vi "Inspect BBM Pad Groups.vi"(7 "Console Log in":refnum<class "Console Log.lvclass">, 8 "error in":errorcluster, 10 "Module Data In":T1={"TBM-TBM"={"Fiducial Image"={"Image Position"=refnum, "Image Reference"=refnum, "Field of View"={"x(mm)"=0.0, "y(mm)"=0.0}}, "Fiducials"=[]}, "TBM-HDI"={"Fiducial Image"={"Image Position"=refnum, "Image Reference"=refnum, "Field of View"={"x(mm)"=0.0, "y(mm)"=0.0}}, "Fiducials"=[]}, "Address Pads"={"Fiducial Image"={"Image Position"=refnum, "Image Reference"=refnum, "Field of View"={"x(mm)"=0.0, "y(mm)"=0.0}}, "Fiducials"=[]}, "HDI Bond Pad References"=[], "BBM Bond Pad References"=[], "HV-HDI"={"Fiducial Image"={"Image Position"=refnum, "Image Reference"=refnum, "Field of View"={"x(mm)"=0.0, "y(mm)"=0.0}}, "Selected Fiducial"={"Fiducial Image Coordinate"=refnum, "Fiducial Source"=enum."Pattern Recognition"}, "fiducial name"=""}, "HV-BBM"={"Fiducial Image"={"Image Position"=refnum, "Image Reference"=refnum, "Field of View"={"x(mm)"=0.0, "y(mm)"=0.0}}, "Selected Fiducial"={"Fiducial Image Coordinate"=refnum, "Fiducial Source"=enum."Pattern Recognition"}, "fiducial name"=""}, "Chuck"=0, "Slot"=0, "Potting Selection"={"HDI Bond Pads"=[TRUE, TRUE, TRUE, TRUE, TRUE, TRUE, TRUE, TRUE, TRUE, TRUE, TRUE, TRUE, TRUE, TRUE, TRUE, TRUE], "BBM Bond Pads"=[TRUE, TRUE, TRUE, TRUE, TRUE, TRUE, TRUE, TRUE, TRUE, TRUE, TRUE, TRUE, TRUE, TRUE, TRUE, TRUE], "TBM Inner"={"Top"=TRUE, "Left"=TRUE, "Bottom"=TRUE, "Right"=TRUE}, "TBM Outer"={"Top"=TRUE, "Left"=TRUE, "Bottom"=TRUE, "Right"=TRUE}, "Address Pads"={"Top"=TRUE, "Bottom"=TRUE}, "High Voltage"={"HDI"=TRUE, "Sensor"=TRUE}}}, 11 "Potting Procedure in":refnum<class "Potting Procedure.lvclass">) -> (0 "error out":errorcluster, 2 "Module Data Out":T1={"TBM-TBM"={"Fiducial Image"={"Image Position"=refnum, "Image Reference"=refnum, "Field of View"={"x(mm)"=0.0, "y(mm)"=0.0}}, "Fiducials"=[]}, "TBM-HDI"={"Fiducial Image"={"Image Position"=refnum, "Image Reference"=refnum, "Field of View"={"x(mm)"=0.0, "y(mm)"=0.0}}, "Fiducials"=[]}, "Address Pads"={"Fiducial Image"={"Image Position"=refnum, "Image Reference"=refnum, "Field of View"={"x(mm)"=0.0, "y(mm)"=0.0}}, "Fiducials"=[]}, "HDI Bond Pad References"=[], "BBM Bond Pad References"=[], "HV-HDI"={"Fiducial Image"={"Image Position"=refnum, "Image Reference"=refnum, "Field of View"={"x(mm)"=0.0, "y(mm)"=0.0}}, "Selected Fiducial"={"Fiducial Image Coordinate"=refnum, "Fiducial Source"=enum."Pattern Recognition"}, "fiducial name"=""}, "HV-BBM"={"Fiducial Image"={"Image Position"=refnum, "Image Reference"=refnum, "Field of View"={"x(mm)"=0.0, "y(mm)"=0.0}}, "Selected Fiducial"={"Fiducial Image Coordinate"=refnum, "Fiducial Source"=enum."Pattern Recognition"}, "fiducial name"=""}, "Chuck"=0, "Slot"=0, "Potting Selection"={"HDI Bond Pads"=[TRUE, TRUE, TRUE, TRUE, TRUE, TRUE, TRUE, TRUE, TRUE, TRUE, TRUE, TRUE, TRUE, TRUE, TRUE, TRUE], "BBM Bond Pads"=[TRUE, TRUE, TRUE, TRUE, TRUE, TRUE, TRUE, TRUE, TRUE, TRUE, TRUE, TRUE, TRUE, TRUE, TRUE, TRUE], "TBM Inner"={"Top"=TRUE, "Left"=TRUE, "Bottom"=TRUE, "Right"=TRUE}, "TBM Outer"={"Top"=TRUE, "Left"=TRUE, "Bottom"=TRUE, "Right"=TRUE}, "Address Pads"={"Top"=TRUE, "Bottom"=TRUE}, "High Voltage"={"HDI"=TRUE, "Sensor"=TRUE}}}, 3 "Potting Procedure out":refnum<class "Potting Procedure.lvclass">, 5 "Console Log out":refnum<class "Console Log.lvclass">)   [LabVIEW 2011, in "Potting Procedure.lvclass"]
uses:
  Potting Procedure.lvclass
  UI Classes/Console Log/Console Log.lvclass
  Type Definitions/Inspect Modules - Module.ctl
  Shared Components/Vec3d Class/Vec3d Class.lvclass
  Shared Components/Utils/Type Definitions/Multi-Fiducial Image.ctl
  Shared Components/Utils/Type Definitions/Physical Image.ctl
  <vilib>/vision/Image Controls.llb/IMAQ Image.ctl
  Shared Components/Utils/Type Definitions/Fiducial with Source.ctl
  Shared Components/Utils/Type Definitions/Fiducial Image.ctl
  Shared Components/WorkTable Class/WorkTable Class.lvclass
  Shared Components/Gantry Class/Gantry Class.lvclass
  Shared Components/Config Manager Class/Type Definitions/Part Type.ctl
  Shared Components/Config Manager Class/Read Geometry Definition 3D.vi
  Shared Components/Config Manager Class/Config Manager Class.lvclass
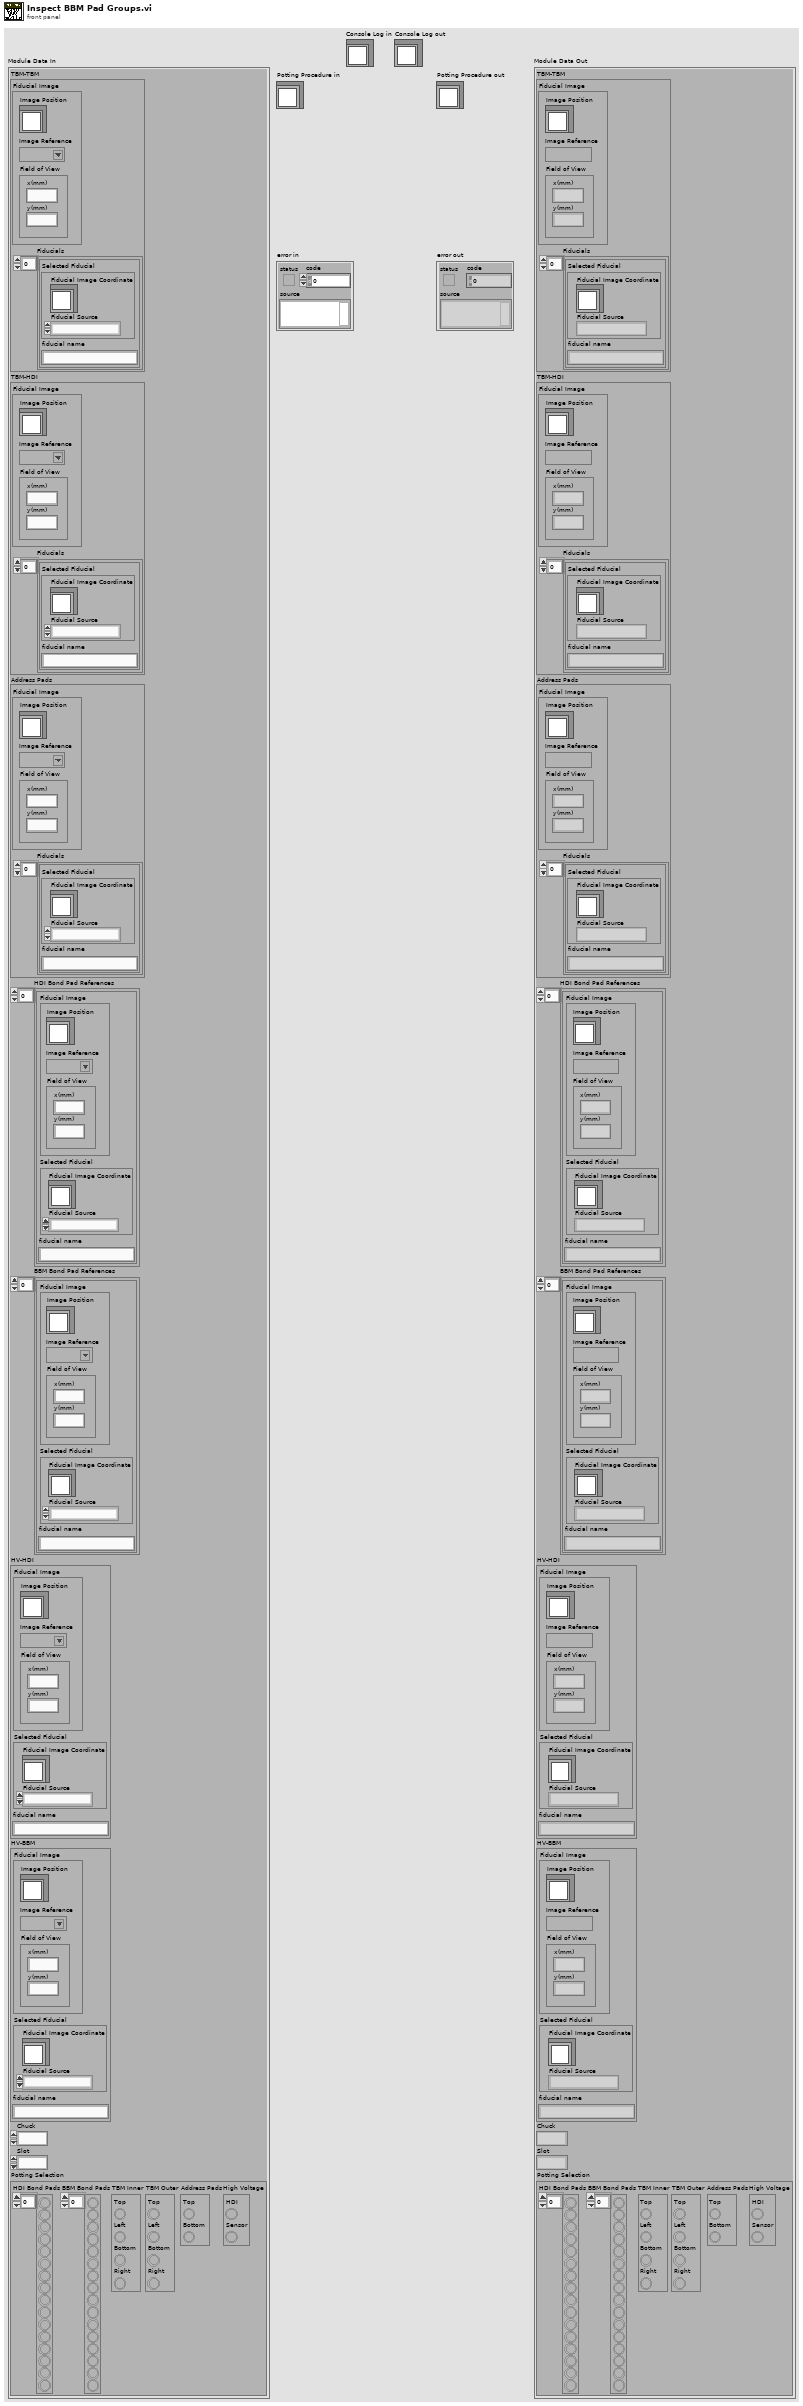
[diagram p1: front panel]
types:
  T1 = typedef "Inspect Modules - Module.ctl" = cluster{"TBM-TBM":T2, "TBM-HDI":T2, "Address Pads":T2, "HDI Bond Pad References":T6[], "BBM Bond Pad References":T6[], "HV-HDI":T6, "HV-BBM":T6, "Chuck":i32, "Slot":i32, "Potting Selection":cluster{"HDI Bond Pads":bool[], "BBM Bond Pads":bool[], "TBM Inner":cluster{"Top":bool, "Left":bool, "Bottom":bool, "Right":bool}, "TBM Outer":cluster{"Top":bool, "Left":bool, "Bottom":bool, "Right":bool}, "Address Pads":cluster{"Top":bool, "Bottom":bool}, "High Voltage":cluster{"HDI":bool, "Sensor":bool}}}
  T2 = typedef "Multi-Fiducial Image.ctl" = cluster{"Fiducial Image":T3, "Fiducials":cluster{"Selected Fiducial":T5, "fiducial name":string}[]}
  T3 = typedef "Physical Image.ctl" = cluster{"Image Position":refnum<class "Vec3d Class.lvclass">, "Image Reference":T4, "Field of View":cluster{"x(mm)":dbl, "y(mm)":dbl}}
  T4 = typedef "IMAQ Image.ctl" = refnum<image>
  T5 = typedef "Fiducial with Source.ctl" = cluster{"Fiducial Image Coordinate":refnum<class "Vec3d Class.lvclass">, "Fiducial Source":enum16{"Pattern Recognition", "User", "Error", "Default"}}
  T6 = typedef "Fiducial Image.ctl" = cluster{"Fiducial Image":T3, "Selected Fiducial":T5, "fiducial name":string}
  T7 = typedef "Part Type.ctl" = enum16{"BBM", "HDI", "GLUERESERVOIR", "STAMP", "WEIGHT"}
  T8 = enum16{"Pattern Recognition", "User", "Error", "Default"}
  T9 = typedef "Worktable_Module Slot.ctl" = cluster{"Slot State":enum16{"Empty", "Unglued", "Stamped", "PartOnTop", "Weighted", "Unpotted", "Potted"}, "BBM Type":enum16{"None", "BBM", "GlassSlide"}, "HDI Type":enum16{"None", "HDI", "Polyimide"}, "Vacuum Channel":u8, "Location/Orientation BBM":T10, "Location/Orientation HDI":T10, "S/N":string}
  T10 = typedef "Position_Orientation.ctl" = cluster{"Center":refnum<class "Vec3d Class.lvclass">, "Orientation":refnum<class "Orient3d Class.lvclass">}
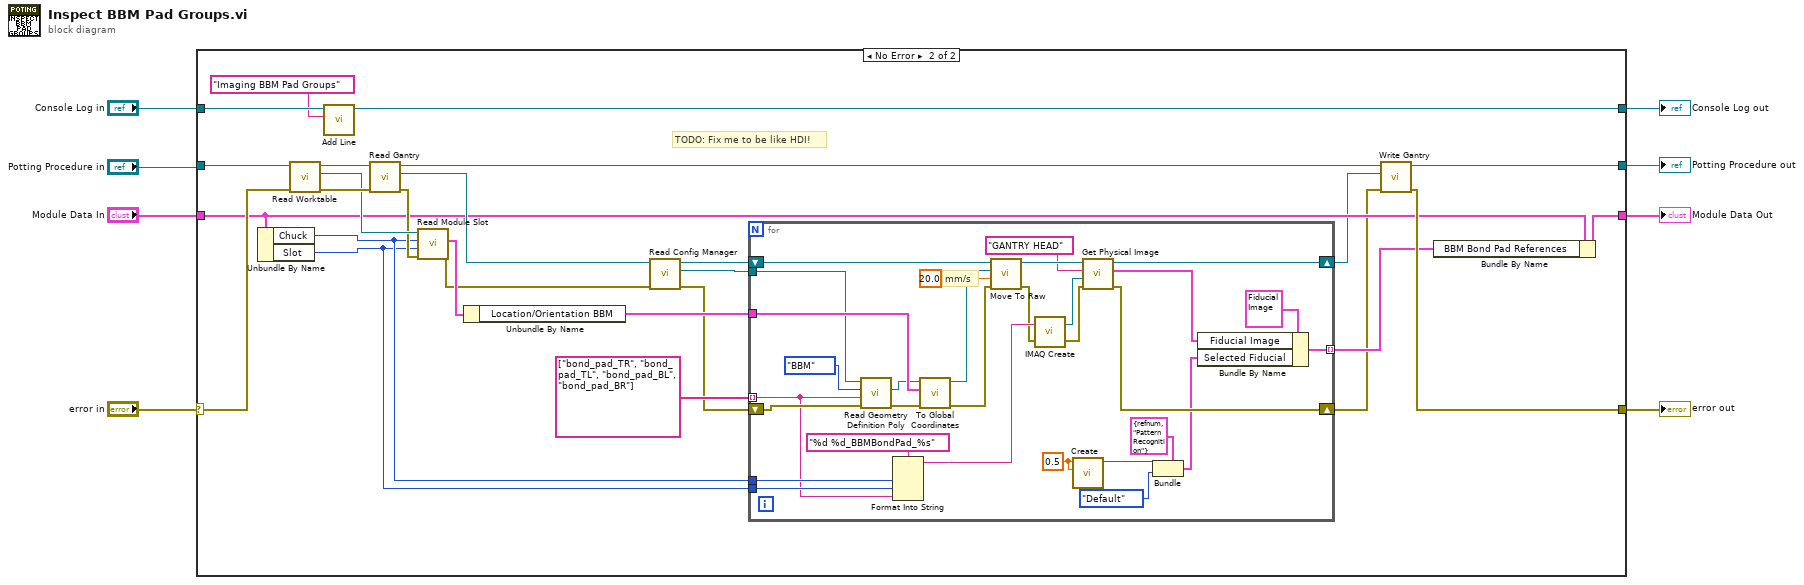
[diagram p0: block diagram]
diagram:
  n1 = case shown="No Error" "error in" {
    selector: "error in" -> [w11 w37]
    tunnel: [w11 w27] -> w6
    tunnel: [w12 w28] -> w5
    tunnel: "Potting Procedure in" -> [w12 w39]
    tunnel: "Module Data In" -> [w10 w26]
    tunnel: [w10 w30] -> w1
    tunnel: "Console Log in" -> [w9 w25]
    tunnel: [w9 w23] -> w3
    frame Error {
    }
    frame No Error {
      # "TODO: Fix me to be like HDI!"
      n2 = Unbundle By Name(w26) -> ("Chuck"=w18:i32, "Slot"=w17:i32)
      n3 = call-dynamic "Read Worktable.vi"("error in"=w37, "Potting Procedure in"=w39) -> ("error out"=w36:errorcluster, "WorkTable out"=w35:refnum<class "WorkTable Class.lvclass">, "Potting Procedure out"=w38:refnum<class "Potting Procedure.lvclass">)  [unwired: 7 in]
      n4 = call "Add Line.vi"("String"="Imaging BBM Pad Groups", "Console Log in"=w25) -> ("Console Log out"=w23:refnum<class "Console Log.lvclass">)  [unwired: 8 in, 1 out]
      n5 = call-dynamic "Read Gantry.vi"("error in (no error)"=w36, "Potting Procedure in"=w38) -> ("error out"=w34:errorcluster, "Gantry"=w32:refnum<class "Gantry Class.lvclass">, "Potting Procedure out"=w29:refnum<class "Potting Procedure.lvclass">)  [unwired: 7 in]
      n6 = call-dynamic "Read Module Slot.vi"("error in"=w34, "slot"=w17, "chuck"=w18, "WorkTable in"=w35) -> ("error out"=w31:errorcluster, "Module Slot"=w33:T9)  [unwired: 5 in, 1 out]
      n7 = Unbundle By Name(w33) -> ("Location/Orientation BBM"=w20:T10)
      n8 = call-dynamic "Read Config Manager.vi"("error in"=w31, "Gantry in"=w32) -> ("error out"=w13:errorcluster, "Config Manager"=w21:refnum<class "Config Manager Class.lvclass">, "Gantry out"=w22:refnum<class "Gantry Class.lvclass">)  [unwired: 7 in]
      n9 = for {
        tunnel: string[] ["bond_pad_TR", "bond_pad_TL", "bond_pad_BL", "bond_pad_BR"] -> [w42] mode=indexing
        tunnel: w20 -> [w69]
        shift-right: [w54] -> w15
        shift-left: w13 -> [w43]
        tunnel: w18 -> [w62]
        tunnel: w17 -> [w61]
        shift-right: [w55] -> w14
        shift-left: w22 -> [w68]
        tunnel: [w46] -> w16 mode=indexing
        tunnel: w21 -> [w45]
        w48 = 0.5 ("X")
        # "mm/s"
        n10 = call-poly "Read Geometry Definition Poly.vi"("error in"=w43, "Feature"=w42, "Part Type"=Part_Type."BBM", "Config Manager in"=w45) -> ("error out"=w40:errorcluster, "Feature Coordinates"=w41:refnum<class "Vec3d Class.lvclass">)  [unwired: 5 in, 1 out]
        n11 = Format Into String(format string="%d %d_BBMBondPad_%s", w62, w61, w42) -> (resulting string=w60:string)  [unwired: 2 in, 1 out]
        n12 = call "To Global Coordinates.vi"("error in"=w40, "Center/Orientation"=w69, "Local Coordinates"=w41) -> ("error out"=w65:errorcluster, "Global Coordinates"=w67:refnum<class "Vec3d Class.lvclass">)  [unwired: 7 in]
        n13 = call-dynamic "Move To Raw.vi"("error in"=w65, "Speed"=20.0, "Destination"=w67, "Gantry in"=w68) -> ("error out"=w59:errorcluster, "Gantry out"=w64:refnum<class "Gantry Class.lvclass">)  [unwired: 6 in]
        n14 = call "IMAQ Create"("Image Name"=w60, "error in (no error)"=w59) -> ("New Image"=w57:T4, "error out"=w58:errorcluster)  [unwired: 3 in]
        n15 = call "Create.vi"("Y"=w48, "X"=w48) -> ("Vec3d Class out"=w49:refnum<class "Vec3d Class.lvclass">)  [unwired: 8 in, 1 out]
        n16 = call-dynamic "Get Physical Image.vi"("error in"=w58, "Image In"=w57, "Camera Name"="GANTRY HEAD", "Gantry in"=w64) -> ("error out"=w54:errorcluster, "Physical Image"=w52:T3, "Gantry out"=w55:refnum<class "Gantry Class.lvclass">)  [unwired: 5 in]
        n17 = Bundle(cluster=T5 {"Fiducial Image Coordinate"=refnum, "Fiducial Source"=enum."Pattern Recognition"} ("Selected Fiducial"), "Fiducial Image Coordinate"=w49, "Fiducial Source"=T8."Default") -> (w50:T5)
        n18 = Bundle By Name(cluster=T6 {"Fiducial Image"={"Image Position"=refnum, "Image Reference"=refnum, "Field of View"={"x(mm)"=0.0, "y(mm)"=0.0}}, "Selected Fiducial"={"Fiducial Image Coordinate"=refnum, "Fiducial Source"=enum."Pattern Recognition"}, "fiducial name"=""} ("Fiducial Image"), "Fiducial Image"=w52, "Selected Fiducial"=w50) -> (w46:T6)
      }
      n19 = call-dynamic "Write Gantry.vi"("error in (no error)"=w15, "Gantry"=w14, "Potting Procedure in"=w29) -> ("error out"=w27:errorcluster, "Potting Procedure out"=w28:refnum<class "Potting Procedure.lvclass">)  [unwired: 7 in]
      n20 = Bundle By Name(cluster=w26, "BBM Bond Pad References"=w16) -> (w30:T1)
    }
  }
  "error out" <- w6
  "Potting Procedure out" <- w5
  "Console Log out" <- w3
  "Module Data Out" <- w1
